vi "NXT_MIDBRAIN Right Wall Follow Behavior Data.vi"(1 "_sensorData":T2={"_irData"={"_irDistance"=0, "_irHeading"=0, "_irTimestamp"=0}, "_batteryVoltage"=0, "_NXTButtonStates"=[FALSE, FALSE, FALSE]}, 2 "Behavior #":i32, 3 "Previous Motor Position":T1={"_rudderCommand"=7, "_propCommand"=7, "_irServoCommand"=7}, 4 "Behavior Weights":T4=[0, 0, 0, 0, 0, 0]) -> (0 "Behavior Output":T5)   [LabVIEW 2012]
uses:
  SKETCHYDELETINGOFALLTHETHINGS/Tugboat/Robo_Programs/behaviorOutput_t.ctl
  SKETCHYDELETINGOFALLTHETHINGS/Tugboat/Robo_Programs/behaviorWeights_t.ctl
  SKETCHYDELETINGOFALLTHETHINGS/Tugboat/Robo_Programs/sensorData_t.ctl
  SKETCHYDELETINGOFALLTHETHINGS/Tugboat/Robo_Programs/irData_t.ctl
  SKETCHYDELETINGOFALLTHETHINGS/Tugboat/Robo_Programs/motorCommands_t.ctl
panel:
  # "L\nE\nF\nT"
  # "C\nE\nN\nT\nE\nR"
  # "R\nI\nG\nH\nT"
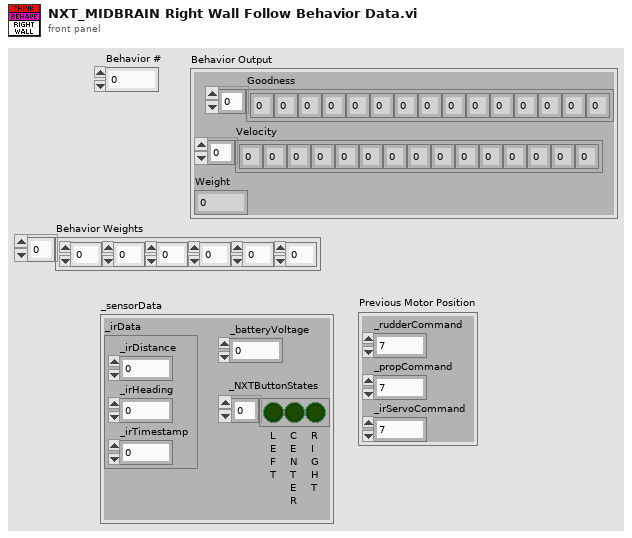
[diagram p1: front panel]
types:
  T1 = typedef "motorCommands_t.ctl" = cluster{"_rudderCommand":i8, "_propCommand":i8, "_irServoCommand":i8}
  T2 = typedef "sensorData_t.ctl" = cluster{"_irData":T3, "_batteryVoltage":i32, "_NXTButtonStates":bool[]}
  T3 = typedef "irData_t.ctl" = cluster{"_irDistance":i32, "_irHeading":i32, "_irTimestamp":u32}
  T4 = typedef "behaviorWeights_t.ctl" = i8[]
  T5 = typedef "behaviorOutput_t.ctl" = cluster{"Goodness":i8[], "Velocity":i8[], "Weight":i8}
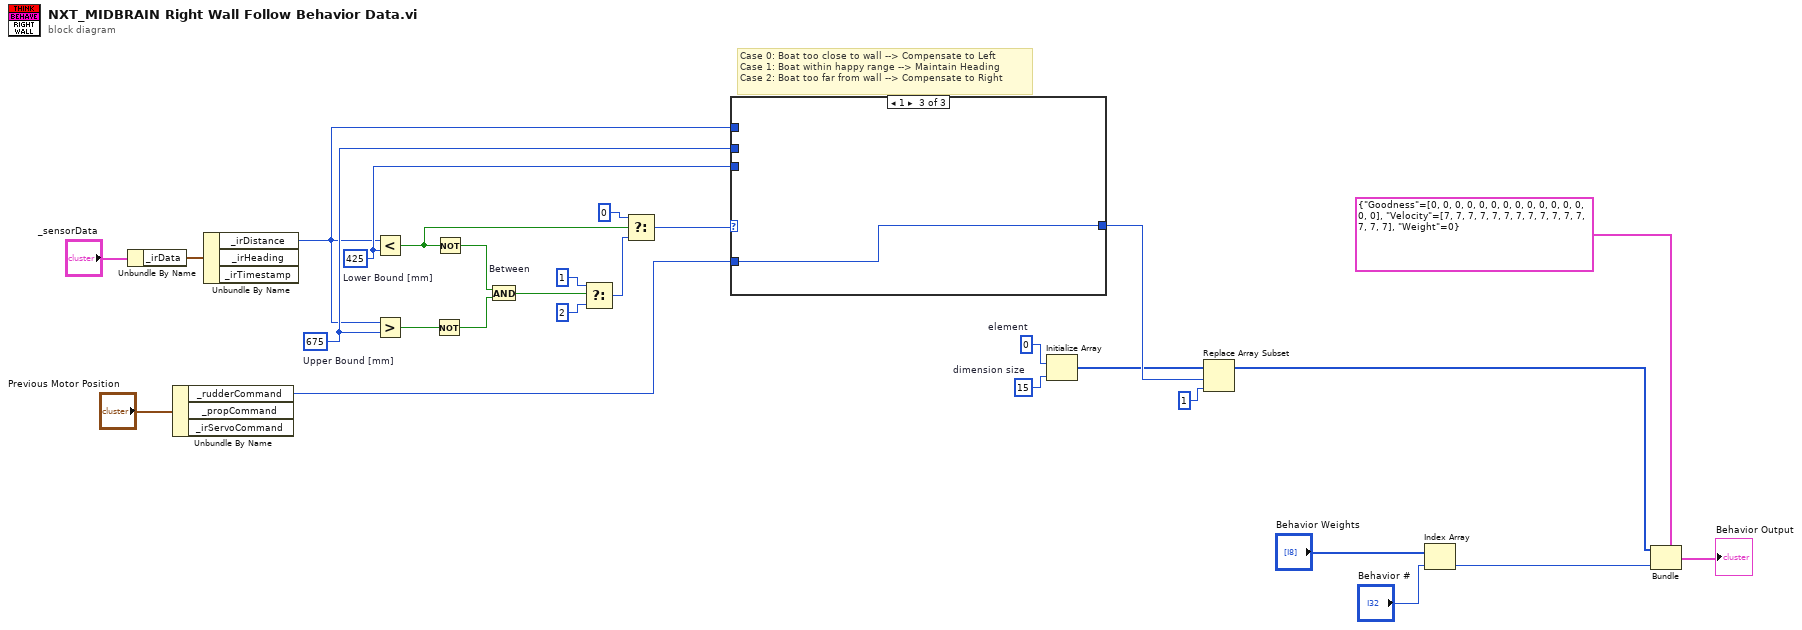
[diagram p0: block diagram]
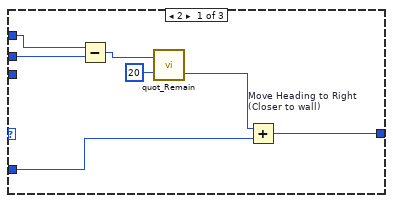
[diagram p2: hidden frame]
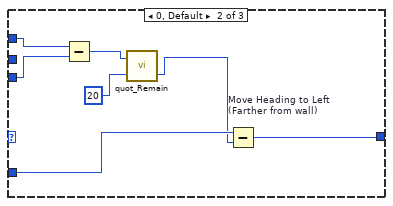
[diagram p3: hidden frame]
diagram:
  w4 = 15  # dimension size
  w5 = i8 0  # element
  w10 = 675  # Upper Bound [mm]
  w9 = 425  # Lower Bound [mm]
  # "Case 0: Boat too close to wall --> Compensate to Left\nCase 1: Boat within happy range --> Maintain Heading\nCase 2: Boat too far from wall --> Compensate to Right"
  n1 = Unbundle By Name("_sensorData") -> ("_irData"=w22:T3)
  n2 = Unbundle By Name("Previous Motor Position") -> ("_rudderCommand"=w11:i8)  [unwired: 2 out]
  n3 = Unbundle By Name(w22) -> ("_irDistance"=w8:i32)  [unwired: 2 out]
  n4 = Less?(x=w8, y=w9) -> (x < y?=w19:bool)
  n5 = Greater?(x=w8, y=w10) -> (0:w16:bool)
  n6 = Not(x=w16) -> (.not. x?=w20:bool)
  n7 = Not(x=w19) -> (.not. x?=w21:bool)
  n8 = And "Between"(x=w21, y=w20) -> (x .and. y?=w18:bool)
  n9 = Select(t=1, s=w18, f=2) -> (s? t:f=w17:i32)
  n10 = Select(t=0, s=w19, f=w17) -> (s? t:f=w1:i32)
  n11 = case shown="1" w1 {
    tunnel: w11 -> [w32 w39 w43]
    tunnel: [w33 w40 w43] -> w7
    tunnel: w10 -> [w34 _ _]
    tunnel: w9 -> [_ w41 _]
    tunnel: w8 -> [w35 w42 _]
    frame 2 {
      n12 = Subtract(x=w35, y=w34) -> (x-y=w29:i8)
      n13 = call <vilib>:"quot_Remain.vi"("y"=i8 20, "x"=w29) -> ("floor(x/y)"=w31:i32)  [unwired: 1 out]
      n14 = Add "Move Heading to Right\n(Closer to wall)"(x=w31, y=w32) -> (x+y=w33:i32)
    }
    frame 0, Default {
      n15 = Subtract(x=w42, y=w41) -> (x-y=w37:i32)
      n16 = call <vilib>:"quot_Remain.vi"("y"=20, "x"=w37) -> ("floor(x/y)"=w38:i32)  [unwired: 1 out]
      n17 = Subtract "Move Heading to Left\n(Farther from wall)"(x=w39, y=w38) -> (x-y=w40:i32)
    }
    frame 1 {
    }
  }
  n18 = Initialize Array(w5, w4) -> (w3:i8[])
  n19 = Replace Array Subset(array=w3, new element=i8 1 ("new element/subarray"), index=w7) -> (w2:i8[])
  n20 = Index Array(array="Behavior Weights", index="Behavior #") -> (element=w24:i8)
  n21 = Bundle(cluster=T5 {"Goodness"=[0, 0, 0, 0, 0, 0, 0, 0, 0, 0, 0, 0, 0, 0, 0], "Velocity"=[7, 7, 7, 7, 7, 7, 7, 7, 7, 7, 7, 7, 7, 7, 7], "Weight"=0} ("Behavior Output"), "Goodness"=w2, "Weight"=w24) -> (→"Behavior Output":T5)  [unwired: 1 in]
